vi "I2C L298P DC Motor Drive.vi"() -> ()   [LabVIEW 2020, in "CTI-Scratchpad.lvlib"]
uses:
  CTI-Scratchpad.lvlib
  CTI/Identity.ctl
  CTI/Error Reporting.ctl
  CTI/GPIO Number.ctl
  CTI/I2C Number.ctl
  CTI-Peripheral/Motor Controller/Base/Direction.ctl
  CTI/Session/Session.lvclass
  CTI-Peripheral/Motor Controller/Grove I2C L298P Motor Drive.lvclass
  CTI/VisaComms/VisaComms.lvclass
  CTI/CTI.lvlib
  CTI-Peripheral/Motor Controller/Base/Motor Controller.lvclass
panel:
  in  "Speed":i16(slide) scale=-100.0..100.0
  in  "Steering":i8(slide) scale=-100.0..100.0
  in  "M2":i16(slide) scale=-255.0..255.0
  in  "M1":i16(slide) scale=-255.0..255.0
  out "loop":i32
  in  "stop":bool
  out "Identity":T1
  in  "Grove Connector":enum16{"I2C0", "I2C1"}(ring)
  out "error out":errorcluster
  in  "Port":refnum<visa-resource-name>="COM6"
  # "https://wiki.seeedstudio.com/Grove-I2C-Motor-Driver-L298P/"
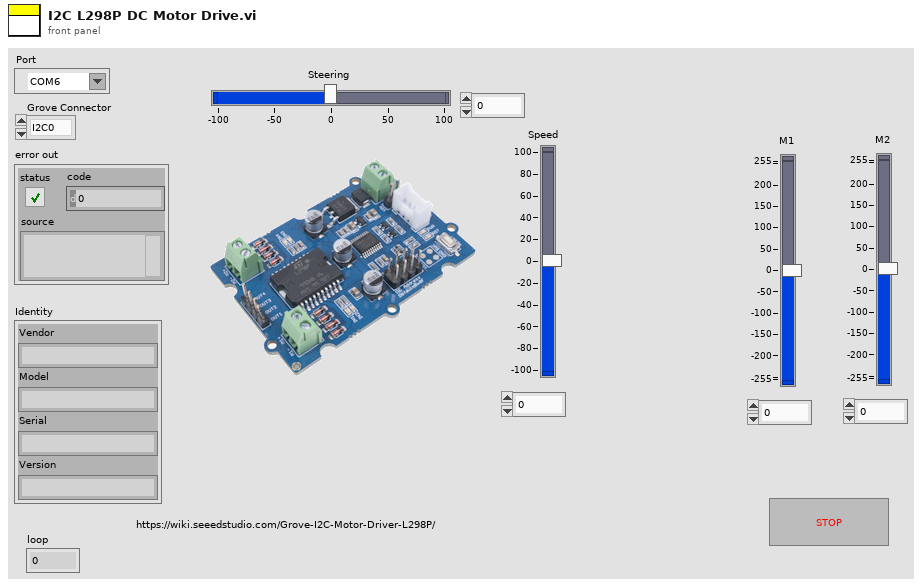
[diagram p1: front panel]
types:
  T1 = typedef "CTI.lvlib/Identity.ctl" = cluster{"Vendor":string, "Model":string, "Serial":string, "Version":string}
  T2 = typedef "CTI.lvlib/Error Reporting.ctl" = enum16{"Minimal", "Moderate", "Full"}
  T3 = typedef "CTI.lvlib/I2C Number.ctl" = i8
  T4 = typedef "CTI.lvlib/GPIO Number.ctl" = i8
  T5 = typedef "CTI-Peripheral.lvlib/Motor Controller.lvclass/Direction.ctl" = enum16{"No Direction - Error", "Clockwise (CW)", "Anti-Clockwise (ACW)"}
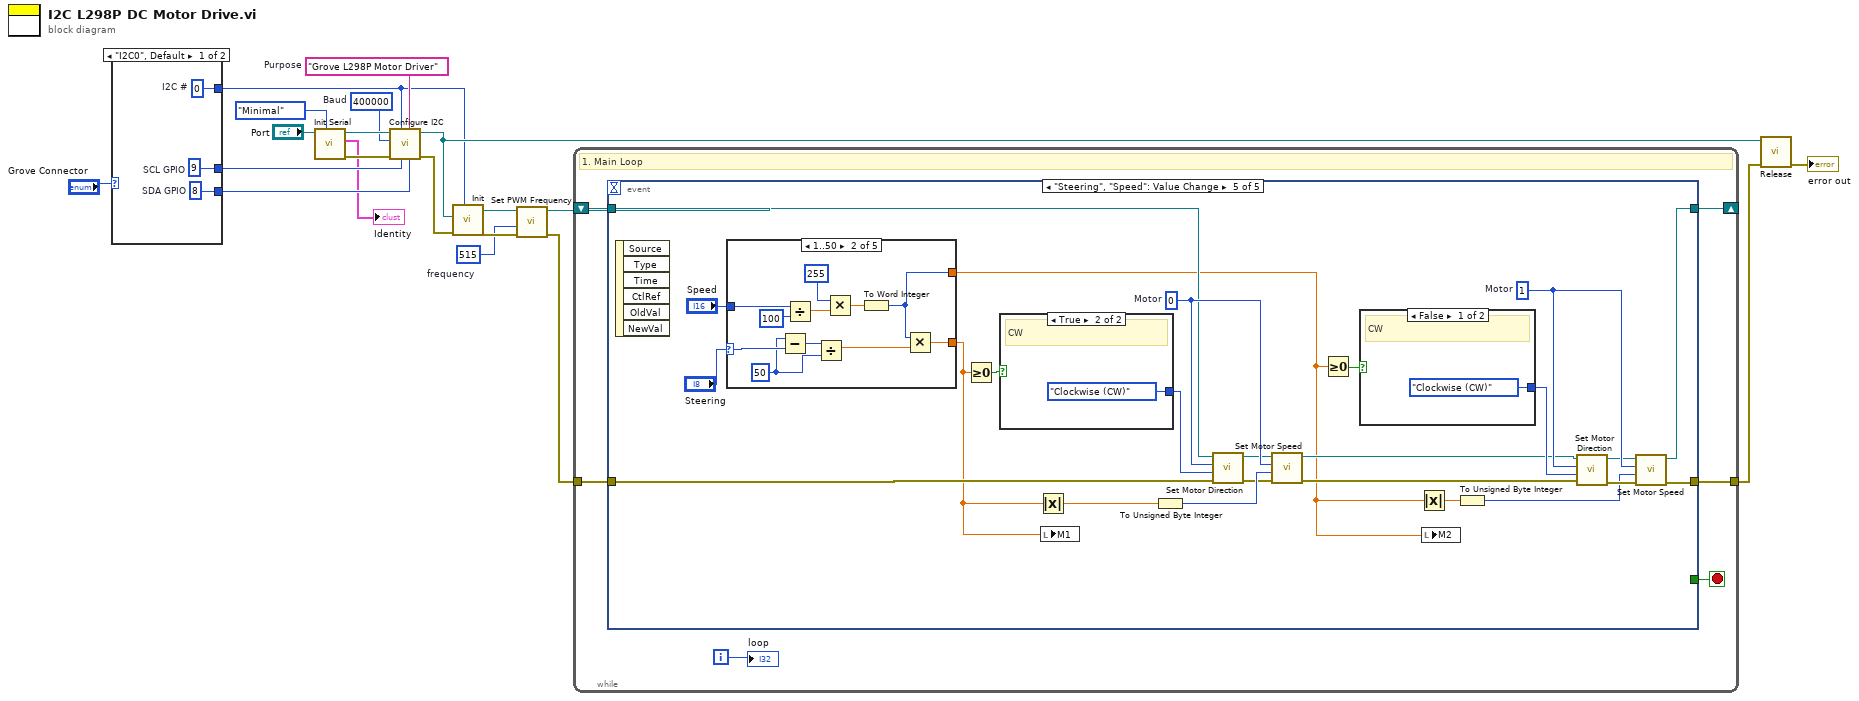
[diagram p0: block diagram]
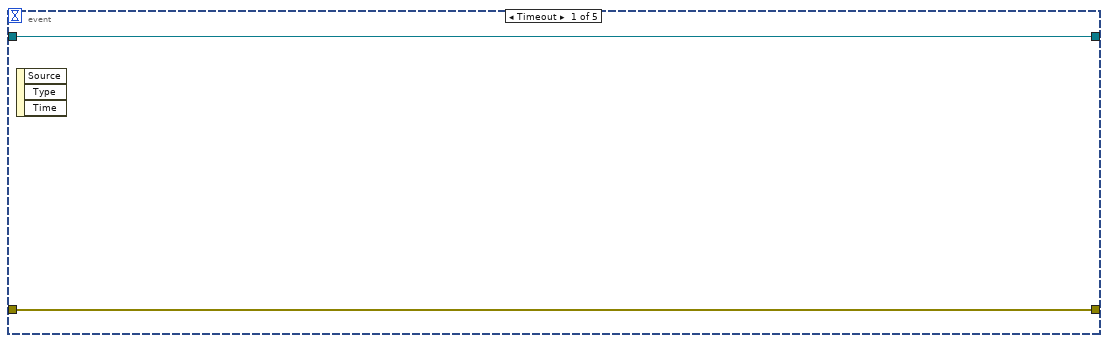
[diagram p2: hidden frame]
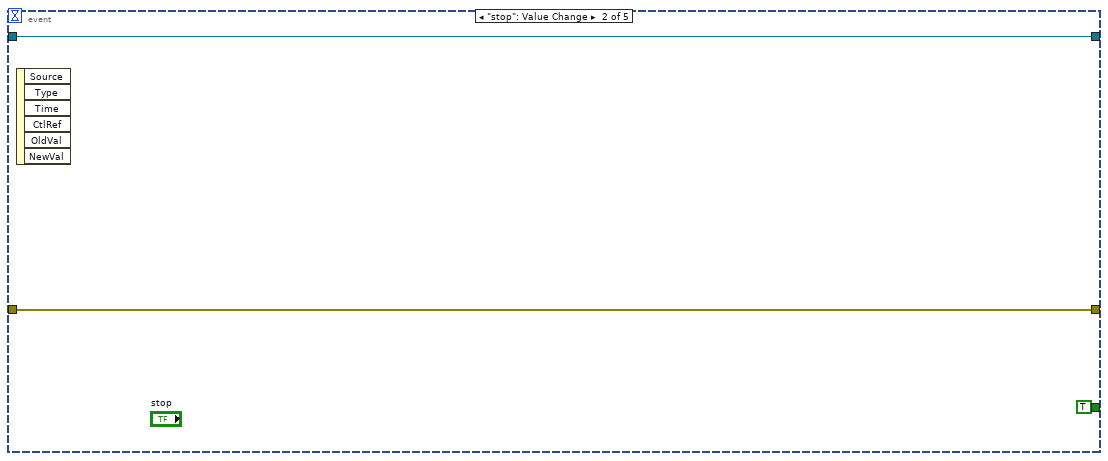
[diagram p3: hidden frame]
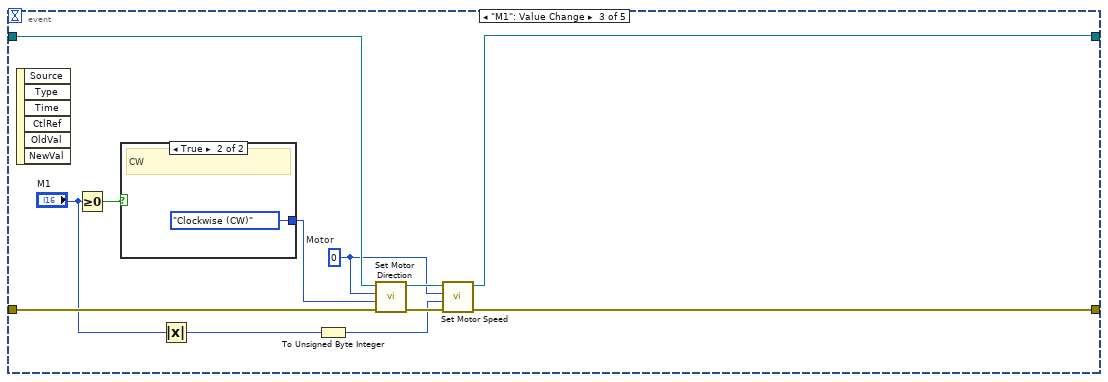
[diagram p4: hidden frame]
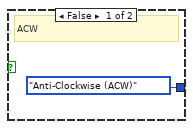
[diagram p5: hidden frame]
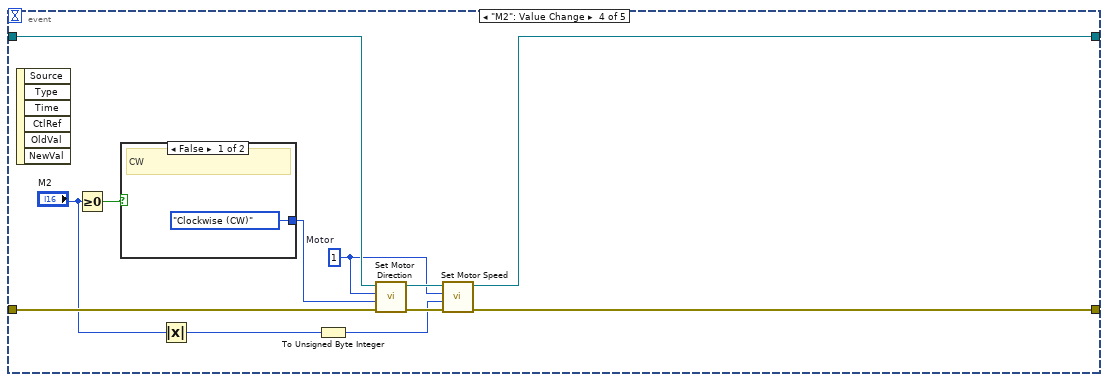
[diagram p6: hidden frame]
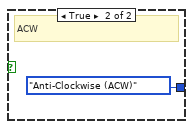
[diagram p7: hidden frame]
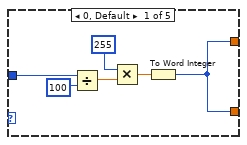
[diagram p8: hidden frame]
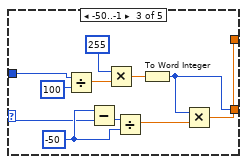
[diagram p9: hidden frame]
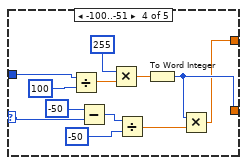
[diagram p10: hidden frame]
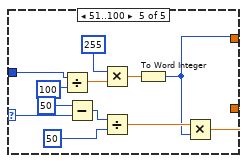
[diagram p11: hidden frame]
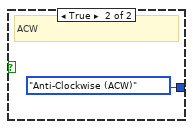
[diagram p12: hidden frame]
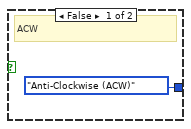
[diagram p13: hidden frame]
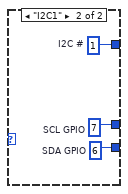
[diagram p14: hidden frame]
diagram:
  w1 = u16 515  # frequency
  w15 = "Grove L298P Motor Driver"  # Purpose
  w16 = u32 400000  # Baud
  n1 = case shown="\"I2C0\", Default" "Grove Connector" {
    tunnel: [w23 w26] -> w13
    tunnel: [w22 w25] -> w12
    tunnel: [w21 w24] -> w7
    frame "I2C0", Default {
      w21 = T3 0  # I2C #
      w22 = T4 8  # SDA GPIO
      w23 = T4 9  # SCL GPIO
    }
    frame "I2C1" {
      w24 = T3 1  # I2C #
      w25 = T4 6  # SDA GPIO
      w26 = T4 7  # SCL GPIO
    }
  }
  n2 = call "Init Serial.vi"("Error Checking (Full)"=Error_Reporting."Minimal", "VISA resource name in"="Port") -> ("error out"=w17:errorcluster, "Identity"=→"Identity":T1, "Session"=w18:refnum<class "Session.lvclass">)  [unwired: 7 in]
  n3 = call "Configure I2C.vi"("SDA GPIO"=w12, "Purpose (\"I2C\")"=w15, "SCL GPIO"=w13, "I2C #"=w7, "error in (no error)"=w17, "Baud"=w16, "Session in"=w18) -> ("error out"=w6:errorcluster, "Session out"=w8:refnum<class "Session.lvclass">)  [unwired: 3 in]
  n4 = call "Init.vi"("I2C #"=w7, "error in (no error)"=w6, "Session In"=w8) -> ("error out"=w4:errorcluster, "Grove I2C L298P Motor Drive Out"=w5:refnum<class "Grove I2C L298P Motor Drive.lvclass">)  [unwired: 7 in]
  n5 = call-dynamic "Set PWM Frequency.vi"("error in (no error)"=w4, "frequency"=w1, "Grove I2C L298P Motor Drive in"=w5) -> ("error out"=w2:errorcluster, "Grove I2C L298P Motor Drive out"=w3:refnum<class "Grove I2C L298P Motor Drive.lvclass">)  [unwired: 7 in]
  n6 = while {
    tunnel: w2 -> [w31]
    tunnel: [w29] -> w10
    shift-right: [w27] -> _
    shift-left: w3 -> [w32]
    i -> [w30]
    stop <- w28 stop-if-true
    # "1. Main Loop"
    n7 = event shown="[4] \"Steering\", \"Speed\": Value Change" {
      selector: _ -> [_ _ _ _ _]
      dyn-events: _ -> [_ _ _ _ _]
      timeout: _ -> [_ _ _ _ _]
      tunnel: w32 -> [w33 w35 w48 w62 w78]
      tunnel: w31 -> [w34 w36 w49 w63 w84]
      tunnel: [w34 w36 w39 w54 w75] -> w29
      tunnel: [_ TRUE _ _ _] -> w28
      tunnel: [w33 w35 w38 w52 w68] -> w27
      event Timeout {
        n8 = event-data() -> ()  [unwired: 1 in, 3 out]
      }
      event "stop": Value Change {
        n9 = event-data() -> ()  [unwired: 1 in, 6 out]
      }
      event "M1": Value Change {
        w43 = u16 0  # Motor
        n10 = event-data() -> ()  [unwired: 1 in, 6 out]
        n11 = Greater Or Equal To 0?(x="M1") -> (x >= 0?=w47:bool)
        n12 = case shown="True" w47 {
          tunnel: [Direction."Anti-Clockwise (ACW)" ("Direction") Direction."Clockwise (CW)" ("Direction")] -> w46
          frame False {
            # "ACW"
          }
          frame True {
            # "CW"
          }
        }
        n13 = Absolute Value(x="M1") -> (abs(x)=w40:i16)
        n14 = To Unsigned Byte Integer(number=w40) -> (unsigned 8bit integer=w41:u8)
        n15 = call-dynamic "Set Motor Direction.vi"("error in (no error)"=w49, "Direction"=w46, "Motor"=w43, "Grove I2C L298P Motor Drive in"=w48) -> ("error out"=w45:errorcluster, "Grove I2C L298P Motor Drive out"=w44:refnum<class "Grove I2C L298P Motor Drive.lvclass">)  [unwired: 6 in]
        n16 = call-dynamic "Set Motor Speed.vi"("error in (no error)"=w45, "Speed"=w41, "Motor"=w43, "Grove I2C L298P Motor Drive in"=w44) -> ("error out"=w39:errorcluster, "Grove I2C L298P Motor Drive out"=w38:refnum<class "Grove I2C L298P Motor Drive.lvclass">)  [unwired: 6 in]
      }
      event "M2": Value Change {
        w57 = u16 1  # Motor
        n17 = event-data() -> ()  [unwired: 1 in, 6 out]
        n18 = Greater Or Equal To 0?(x="M2") -> (x >= 0?=w61:bool)
        n19 = case shown="False" w61 {
          tunnel: [Direction."Clockwise (CW)" ("Direction") Direction."Anti-Clockwise (ACW)" ("Direction")] -> w60
          frame False {
            # "CW"
          }
          frame True {
            # "ACW"
          }
        }
        n20 = Absolute Value(x="M2") -> (abs(x)=w55:i16)
        n21 = To Unsigned Byte Integer(number=w55) -> (unsigned 8bit integer=w56:u8)
        n22 = call-dynamic "Set Motor Direction.vi"("error in (no error)"=w63, "Direction"=w60, "Motor"=w57, "Grove I2C L298P Motor Drive in"=w62) -> ("error out"=w59:errorcluster, "Grove I2C L298P Motor Drive out"=w58:refnum<class "Grove I2C L298P Motor Drive.lvclass">)  [unwired: 6 in]
        n23 = call-dynamic "Set Motor Speed.vi"("error in (no error)"=w59, "Speed"=w56, "Motor"=w57, "Grove I2C L298P Motor Drive in"=w58) -> ("error out"=w54:errorcluster, "Grove I2C L298P Motor Drive out"=w52:refnum<class "Grove I2C L298P Motor Drive.lvclass">)  [unwired: 6 in]
      }
      event "Steering", "Speed": Value Change {
        w83 = u16 1  # Motor
        w85 = u16 0  # Motor
        n24 = event-data() -> ()  [unwired: 1 in, 6 out]
        n25 = case shown="1..50" "Steering" {
          selector: "Steering" -> [_ w98 w108 w121 w133]
          tunnel: "Speed" -> [w95 w102 w113 w127 w137]
          tunnel: [w90 w99 w111 w123 w130] -> w72
          tunnel: [w90 w100 w110 w118 w135] -> w66
          frame 0, Default {
            n26 = Divide(x=w95, y=u8 100) -> (x/y=w93:dbl)
            n27 = Multiply(x=i16 255 ("Value (Signaling)"), y=w93) -> (x*y=w92:dbl)
            n28 = To Word Integer(number=w92) -> (16bit integer=w90:i16)
          }
          frame 1..50 {
            w97 = i8 50 ("x")
            n29 = Subtract(x=w97, y=w98) -> (x-y=w96:i8)
            n30 = Divide(x=w102, y=u8 100) -> (x/y=w105:dbl)
            n31 = Divide(x=w96, y=w97) -> (x/y=w101:dbl)
            n32 = Multiply(x=i16 255 ("Value (Signaling)"), y=w105) -> (x*y=w104:dbl)
            n33 = To Word Integer(number=w104) -> (16bit integer=w100:i16)
            n34 = Multiply(x=w100, y=w101) -> (x*y=w99:dbl)
          }
          frame -50..-1 {
            w109 = i8 -50 ("x")
            n35 = Divide(x=w113, y=u8 100) -> (x/y=w116:dbl)
            n36 = Subtract(x=w109, y=w108) -> (x-y=w107:i8)
            n37 = Multiply(x=i16 255 ("Value (Signaling)"), y=w116) -> (x*y=w115:dbl)
            n38 = Divide(x=w107, y=w109) -> (x/y=w112:dbl)
            n39 = To Word Integer(number=w115) -> (16bit integer=w111:i16)
            n40 = Multiply(x=w111, y=w112) -> (x*y=w110:dbl)
          }
          frame -100..-51 {
            n41 = Divide(x=w127, y=u8 100) -> (x/y=w129:dbl)
            n42 = Subtract(x=i8 -50, y=w121) -> (x-y=w120:i8)
            n43 = Multiply(x=i16 255 ("Value (Signaling)"), y=w129) -> (x*y=w128:dbl)
            n44 = Divide(x=w120, y=i8 -50 ("x")) -> (x/y=w124:dbl)
            n45 = To Word Integer(number=w128) -> (16bit integer=w123:i16)
            n46 = Multiply(x=w123, y=w124) -> (x*y=w118:dbl)
          }
          frame 51..100 {
            n47 = Divide(x=w137, y=u8 100) -> (x/y=w140:dbl)
            n48 = Subtract(x=i8 50, y=w133) -> (x-y=w132:i8)
            n49 = Multiply(x=i16 255 ("Value (Signaling)"), y=w140) -> (x*y=w139:dbl)
            n50 = Divide(x=w132, y=i8 50 ("x")) -> (x/y=w136:dbl)
            n51 = To Word Integer(number=w139) -> (16bit integer=w135:i16)
            n52 = Multiply(x=w136, y=w135) -> (x*y=w130:dbl)
          }
        }
        n53 = Greater Or Equal To 0?(x=w72) -> (x >= 0?=w88:bool)
        n54 = case shown="True" w88 {
          tunnel: [Direction."Anti-Clockwise (ACW)" ("Direction") Direction."Clockwise (CW)" ("Direction")] -> w87
          frame False {
            # "ACW"
          }
          frame True {
            # "CW"
          }
        }
        n55 = Absolute Value(x=w72) -> (abs(x)=w86:dbl)
        n56 = local write "M1"(w72) -> ()
        n57 = To Unsigned Byte Integer(number=w86) -> (unsigned 8bit integer=w74:u8)
        n58 = call-dynamic "Set Motor Direction.vi"("error in (no error)"=w84, "Direction"=w87, "Motor"=w85, "Grove I2C L298P Motor Drive in"=w78) -> ("error out"=w71:errorcluster, "Grove I2C L298P Motor Drive out"=w70:refnum<class "Grove I2C L298P Motor Drive.lvclass">)  [unwired: 6 in]
        n59 = call-dynamic "Set Motor Speed.vi"("error in (no error)"=w71, "Speed"=w74, "Motor"=w85, "Grove I2C L298P Motor Drive in"=w70) -> ("error out"=w80:errorcluster, "Grove I2C L298P Motor Drive out"=w69:refnum<class "Grove I2C L298P Motor Drive.lvclass">)  [unwired: 6 in]
        n60 = Greater Or Equal To 0?(x=w66) -> (x >= 0?=w79:bool)
        n61 = case shown="False" w79 {
          tunnel: [Direction."Clockwise (CW)" ("Direction") Direction."Anti-Clockwise (ACW)" ("Direction")] -> w77
          frame False {
            # "CW"
          }
          frame True {
            # "ACW"
          }
        }
        n62 = Absolute Value(x=w66) -> (abs(x)=w76:dbl)
        n63 = local write "M2"(w66) -> ()
        n64 = To Unsigned Byte Integer(number=w76) -> (unsigned 8bit integer=w73:u8)
        n65 = call-dynamic "Set Motor Direction.vi"("error in (no error)"=w80, "Direction"=w77, "Motor"=w83, "Grove I2C L298P Motor Drive in"=w69) -> ("error out"=w81:errorcluster, "Grove I2C L298P Motor Drive out"=w82:refnum<class "Grove I2C L298P Motor Drive.lvclass">)  [unwired: 6 in]
        n66 = call-dynamic "Set Motor Speed.vi"("error in (no error)"=w81, "Speed"=w73, "Motor"=w83, "Grove I2C L298P Motor Drive in"=w82) -> ("error out"=w75:errorcluster, "Grove I2C L298P Motor Drive out"=w68:refnum<class "Grove I2C L298P Motor Drive.lvclass">)  [unwired: 6 in]
      }
    }
    "loop" <- w30
  }
  n67 = call-dynamic "Release.vi"("error in (no error)"=w10, "Session in"=w8) -> ("error out"=→"error out":errorcluster)  [unwired: 9 in]
